vi "FTW-Endpoint-Core-Poll.vi"(0 "FTW Endpoint":refnum<class "FTW-Endpoint.lvclass">, 5 "Check for Incoming Messages?":bool, 7 "Check for Outgoing Messages?":bool, 9 "Timeout":i32 format="%dmsec", 11 "error in":errorcluster) -> (4 "FTW Endpoint out":refnum<class "FTW-Endpoint.lvclass">, 6 "Incoming Message Available":bool, 8 "Outgoing Message Available":bool, 15 "error out":errorcluster)   [LabVIEW 2012, in "FTW-Actor.lvlib" / "FTW-Endpoint.lvclass"]
uses:
  FTW-Endpoint.lvclass
  FTW-Endpoint.lvclass/FTW-Endpoint.ctl
panel:
  # "Inputs"
  # "Outputs"
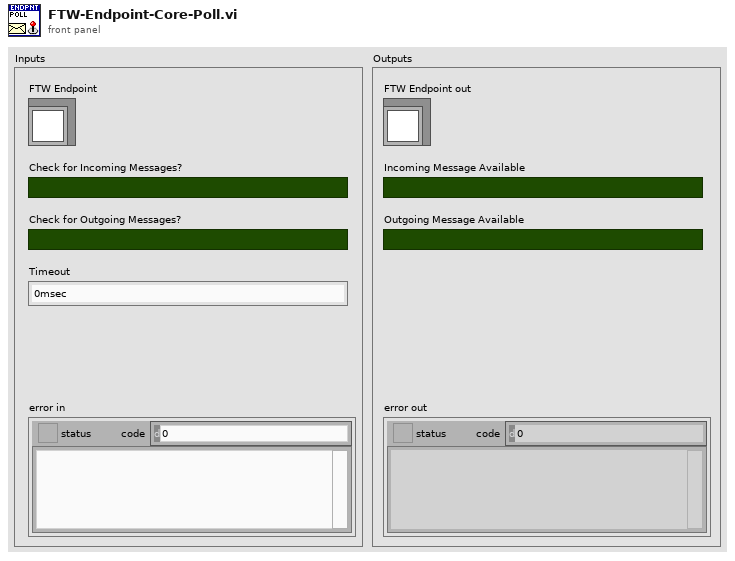
[diagram p1: front panel]
types:
  T1 = cluster{"SocketID":i32, "Events to Check":i16, "Return Value":i16}
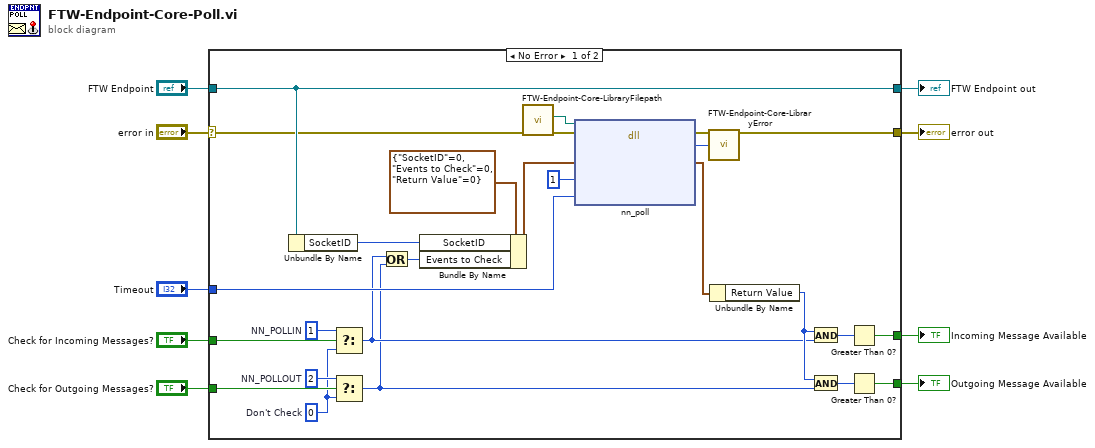
[diagram p0: block diagram]
diagram:
  n1 = case shown="No Error" "error in" {
    selector: "error in" -> [w18 w36]
    tunnel: "FTW Endpoint" -> [w19 w37]
    tunnel: "Timeout" -> [w31 _]
    tunnel: [w26 w36] -> w7
    tunnel: [w22 _] -> w6
    tunnel: [w20 _] -> w5
    tunnel: [w19 w37] -> w4
    tunnel: "Check for Incoming Messages?" -> [w16 _]
    tunnel: "Check for Outgoing Messages?" -> [w11 _]
    frame No Error {
      w10 = i16 0  # Don't Check
      w13 = i16 2  # NN_POLLOUT
      w15 = i16 1  # NN_POLLIN
      n2 = Unbundle By Name(w19) -> ("SocketID"=w17:i64)
      n3 = Select(t=w15, s=w16, f=w10) -> (s? t:f=w14:i16)
      n4 = Select(t=w13, s=w11, f=w10) -> (s? t:f=w12:i16)
      n5 = Or(x=w14, y=w12) -> (x .or. y?=w24:i16)
      n6 = Bundle By Name(cluster=T1 {"SocketID"=0, "Events to Check"=0, "Return Value"=0} ("fds"), "SocketID"=w17, "Events to Check"=w24) -> (w32:T1)
      n7 = call "FTW-Endpoint-Core-LibraryFilepath.vi"("error in"=w18) -> ("error out"=w30:errorcluster, "Library Filepath"=w29:path)  [unwired: 8 in, 1 out]
      n8 = dll-call lib="?" fn="nn_poll"(path in=w29, error in=w30, "File Descriptors"=w32, "Num File Descriptors"=1, "Timeout"=w31) -> (error out=w27:errorcluster, "Return Value"=w28:i64, "File Descriptors"=w25:T1)  [unwired: 3 in, 1 out]
      n9 = call "FTW-Endpoint-Core-LibraryError.vi"("error in"=w27, "Return Value"=w28) -> ("error out"=w26:errorcluster)  [unwired: 13 in]
      n10 = Unbundle By Name(w25) -> ("Return Value"=w23:i16)
      n11 = And(x=w23, y=w14) -> (x .and. y?=w33:i16)
      n12 = And(x=w23, y=w12) -> (x .and. y?=w21:i16)
      n13 = Greater Than 0?(x=w33) -> (x > 0?=w22:bool)
      n14 = Greater Than 0?(x=w21) -> (x > 0?=w20:bool)
    }
    frame Error {
    }
  }
  "error out" <- w7
  "FTW Endpoint out" <- w4
  "Incoming Message Available" <- w6
  "Outgoing Message Available" <- w5
